vi "CRYBark_Loudness.vi"() -> ()   [LabVIEW 2013]
panel:
  out "XY Graph 3":cluster{dbl[], dbl[]}(graph) caption="Stimulus_Ear_Graph"
  out "XY Graph 2":cluster{dbl[], dbl[]}(graph) caption="Stimulus_Ear_Graph"
  in  "Numeric":dbl
  out "XY Graph":cluster{dbl[], dbl[]}(graph) caption="Stimulus_Ear_Graph"
  out "Loudness(sone)":dbl[](array[numeric])
  out "Loudness":dbl
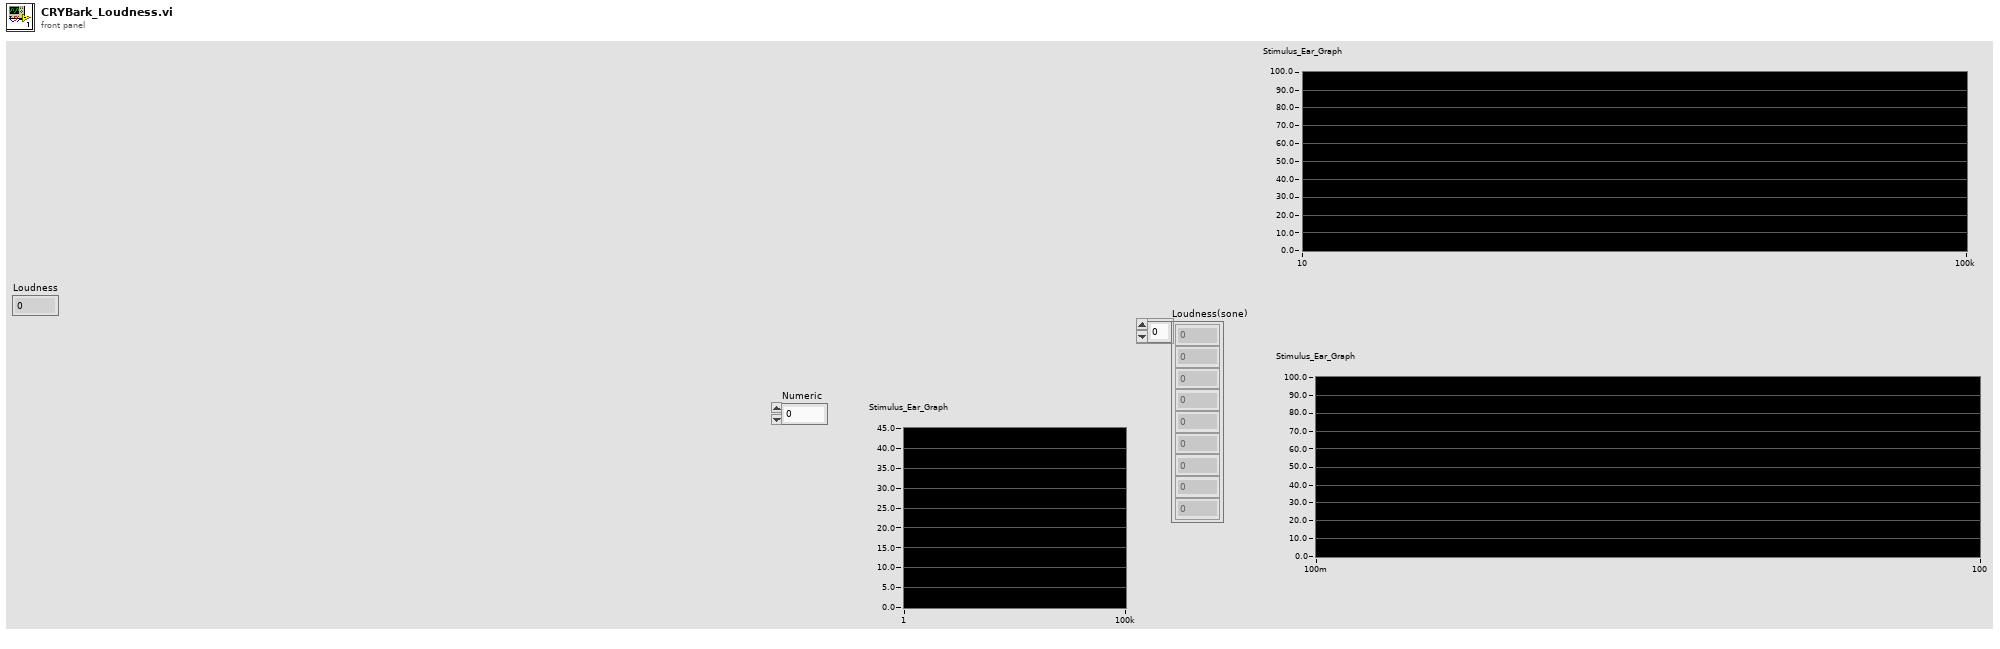
[diagram p1: front panel]
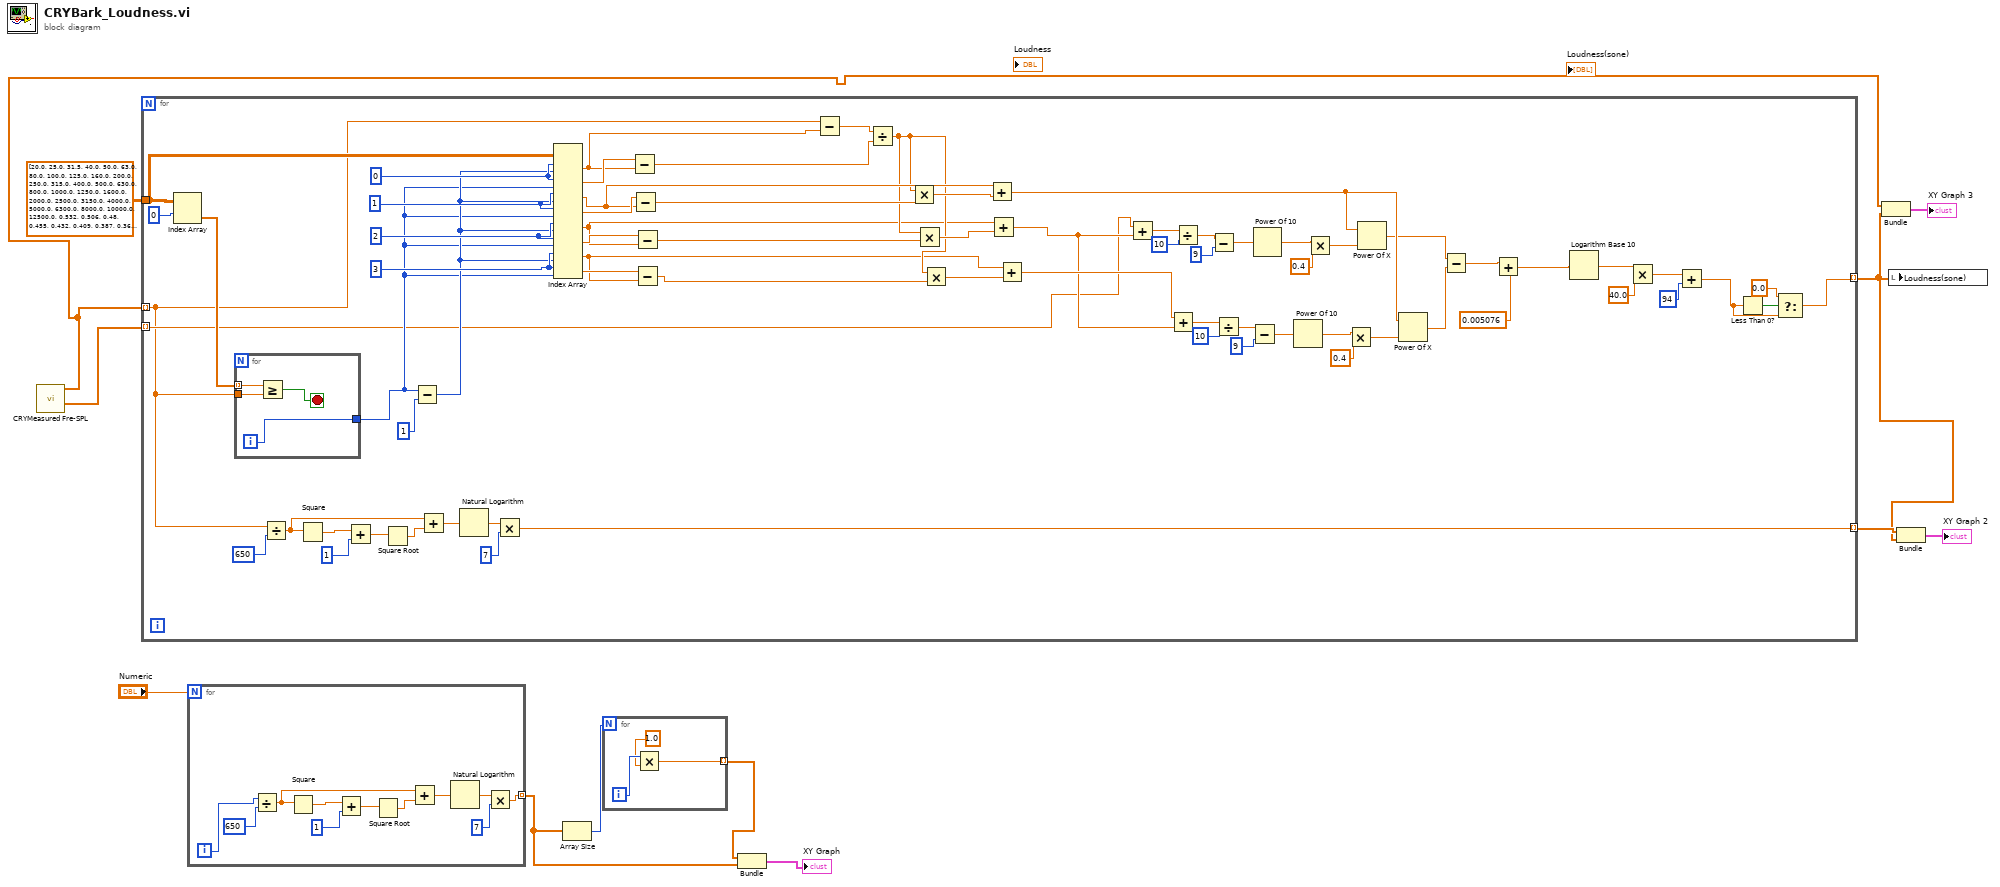
[diagram p0: block diagram]
diagram:
  n1 = call "CRYMeasured Fre-SPL.vi"() -> ("measured frequency"=w1:dbl[], "measured SPL"=w4:dbl[])  [unwired: 8 in]
  n2 = for {
    tunnel: dbl[][] [[20.0, 25.0, 31.5, 40.0, 50.0, 63.0, 80.0, 100.0, 125.0, 160.0, 200.0, 250.0, 315.0, 400.0, 500.0, 630.0, 800.0, 1000.0, 1250.0, 1600.0, 2000.0, 2500.0, 3150.0, 4000.0, 5000.0, 6300.0, 8000.0, 10000.0, 12500.0], [0.532, 0.506, 0.48, 0.455, 0.432, 0.409, 0.387, 0.367, 0.349, 0.33, 0.315, 0.301, 0.288, 0.276, 0.267, 0.259, 0.253, 0.25, 0.246, 0.244, 0.243, 0.243, 0.243, 0.242, 0.242, 0.245, 0.254, 0.271, 0.301], [-31.6, -27.2, -23.0, -19.1, -15.9, -13.0, -10.3, -8.1, -6.2, -4.5, -3.1, -2.0, -1.1, -0.4, 0.0, 0.3, 0.5, 0.0, -2.7, -4.1, -1.0, 1.7, 2.5, 1.2, -2.1, -7.1, -11.2, -10.7, -3.1], [78.5, 68.7, 59.5, 51.1, 44.0, 37.5, 31.5, 26.5, 22.1, 17.9, 14.4, 11.4, 8.6, 6.2, 4.4, 3.0, 2.2, 2.4, 3.5, 1.7, -1.3, -4.2, -6.0, -5.4, -1.5, 6.0, 12.6, 13.9, 12.3]] -> [w81]
    tunnel: w1 -> [w18] mode=indexing
    tunnel: w4 -> [w28] mode=indexing
    tunnel: [w13] -> w2 mode=indexing
    tunnel: [w17] -> w5 mode=indexing
    w76 = 3
    w77 = 2
    w78 = 1
    w79 = 0
    n3 = Index Array(array=w81, index (row)=0) -> (element=w82:dbl[])  [unwired: 1 in]
    n4 = for {
      tunnel: w82 -> [w87] mode=indexing
      tunnel: w18 -> [w86]
      tunnel: [w84] -> w74
      i -> [w84]
      stop <- w85 stop-if-true
      n5 = Greater Or Equal?(x=w87, y=w86) -> (x >= y?=w85:bool)
    }
    n6 = Divide(x=w18, y=650) -> (x/y=w24:dbl)
    n7 = Square(x=w24) -> (x^2=w20:dbl)
    n8 = Add(x=w20, y=1) -> (x+y=w22:dbl)
    n9 = Square Root(x=w22) -> (sqrt(x)=w23:dbl)
    n10 = Subtract(x=w74, y=1) -> (x-y=w75:i32)
    n11 = Add(x=w24, y=w23) -> (x+y=w25:dbl)
    n12 = Natural Logarithm(1:w25) -> (0:w26:dbl)
    n13 = Multiply(x=w26, y=7) -> (x*y=w17:dbl)
    n14 = Index Array(array=w81, index (row) #1=w79, index (col) #1=w75, index (row) #2=w79, index (col) #2=w74, index (row) #3=w78, index (col) #3=w75, index (row) #4=w78, index (col) #4=w74, index (row) #5=w77, index (col) #5=w75, index (row) #6=w77, index (col) #6=w74, index (row) #7=w76, index (col) #7=w75, index (row) #8=w76, index (col) #8=w74) -> (element #1=w69:dbl, element #2=w73:dbl, element #3=w62:dbl, element #4=w72:dbl, element #5=w59:dbl, element #6=w71:dbl, element #7=w58:dbl, element #8=w70:dbl)
    n15 = Subtract(x=w73, y=w69) -> (x-y=w67:dbl)
    n16 = Subtract(x=w72, y=w62) -> (x-y=w66:dbl)
    n17 = Subtract(x=w71, y=w59) -> (x-y=w65:dbl)
    n18 = Subtract(x=w70, y=w58) -> (x-y=w64:dbl)
    n19 = Subtract(x=w18, y=w69) -> (x-y=w68:dbl)
    n20 = Divide(x=w68, y=w67) -> (x/y=w60:dbl)
    n21 = Multiply(x=w60, y=w66) -> (x*y=w63:dbl)
    n22 = Multiply(x=w60, y=w65) -> (x*y=w61:dbl)
    n23 = Multiply(x=w60, y=w64) -> (x*y=w57:dbl)
    n24 = Add(x=w62, y=w63) -> (x+y=w40:dbl)
    n25 = Add(x=w59, y=w61) -> (x+y=w38:dbl)
    n26 = Add(x=w58, y=w57) -> (x+y=w39:dbl)
    n27 = Add(x=w28, y=w38) -> (x+y=w56:dbl)
    n28 = Add(x=w39, y=w38) -> (x+y=w41:dbl)
    n29 = Divide(x=w56, y=10) -> (x/y=w54:dbl)
    n30 = Subtract(x=w54, y=9) -> (x-y=w52:dbl)
    n31 = Divide(x=w41, y=10) -> (x/y=w43:dbl)
    n32 = Subtract(x=w43, y=9) -> (x-y=w45:dbl)
    n33 = Power Of 10(x=w52) -> (10^x=w51:dbl)
    n34 = Power Of 10(x=w45) -> (10^x=w46:dbl)
    n35 = Multiply(x=w51, y=0.4) -> (x*y=w49:dbl)
    n36 = Multiply(x=w46, y=0.4) -> (x*y=w48:dbl)
    n37 = Power Of X(1:w49, 2:w40) -> (0:w37:dbl)
    n38 = Power Of X(1:w48, 2:w40) -> (0:w36:dbl)
    n39 = Subtract(x=w37, y=w36) -> (x-y=w35:dbl)
    n40 = Add(x=w35, y=0.005076) -> (x+y=w33:dbl)
    n41 = Logarithm Base 10(1:w33) -> (0:w31:dbl)
    n42 = Multiply(x=w31, y=40.0) -> (x*y=w30:dbl)
    n43 = Add(x=w30, y=94) -> (x+y=w14:dbl)
    n44 = Less Than 0?(x=w14) -> (x < 0?=w16:bool)
    n45 = Select(t=0.0, s=w16, f=w14) -> (s? t:f=w13:dbl)
  }
  n46 = for {
    N: "Numeric" -> [_]
    tunnel: [w88] -> w8 mode=indexing
    i -> [w97]
    n47 = Divide(x=w97, y=650) -> (x/y=w92:dbl)
    n48 = Square(x=w92) -> (x^2=w96:dbl)
    n49 = Add(x=w96, y=1) -> (x+y=w94:dbl)
    n50 = Square Root(x=w94) -> (sqrt(x)=w93:dbl)
    n51 = Add(x=w92, y=w93) -> (x+y=w91:dbl)
    n52 = Natural Logarithm(1:w91) -> (0:w90:dbl)
    n53 = Multiply(x=w90, y=7) -> (x*y=w88:dbl)
  }
  n54 = Array Size(array=w8) -> (size(s)=w10:i32)
  n55 = for {
    N: w10 -> [_]
    tunnel: [w99] -> w9 mode=indexing
    i -> [w101]
    n56 = Multiply(x=w101, y=1.0 ("Numeric 3")) -> (x*y=w99:dbl)
  }
  n57 = Bundle(w9, w8) -> (→"XY Graph":cluster{dbl[], dbl[]})  [unwired: 1 out]
  n58 = Bundle("measured frequency"=w1, w2) -> (→"XY Graph 3":cluster{"measured frequency":dbl[], dbl[]})  [unwired: 1 out]
  n59 = local write "Loudness(sone)"(w2) -> ()
  n60 = Bundle(w5, w2) -> (→"XY Graph 2":cluster{dbl[], dbl[]})  [unwired: 1 out]
